vi "Load and Validate_Extract Number.vi"(11 "String":string) -> (3 "Numeric":i32)   [LabVIEW 2020, in "ProjectBuilder.lvlib"]
uses:
  ProjectBuilder.lvlib
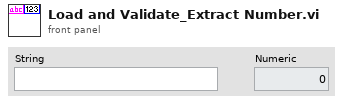
[diagram p1: front panel]
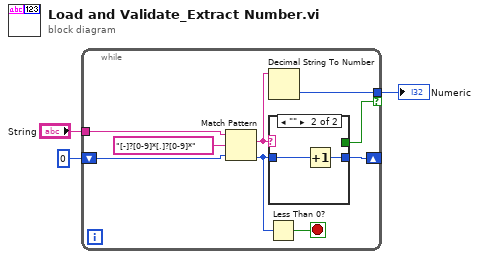
[diagram p0: block diagram]
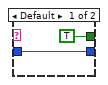
[diagram p2: hidden frame]
diagram:
  n1 = while {
    tunnel: [w12] -> w3 if=w7
    tunnel: "String" -> [w10]
    shift-right: [w6] -> _
    shift-left: 0 -> [w9]
    stop <- w4 stop-if-true
    n2 = Match Pattern(string=w10, regular expression="[-]?[0-9]*[.]?[0-9]*", offset (0)=w9) -> (match substring=w8:string, offset past match=w5:i32)  [unwired: 2 out]
    n3 = Less Than 0?(x=w5) -> (x < 0?=w4:bool)
    n4 = Decimal String To Number(string=w8) -> (number=w12:i32)  [unwired: 2 in, 1 out]
    n5 = case shown="\"\"" w8 {
      tunnel: [w14 w15] -> w6
      tunnel: [TRUE _] -> w7
      tunnel: w5 -> [w14 w16]
      frame Default {
      }
      frame "" {
        n6 = Increment(x=w16) -> (x+1=w15:i32)
      }
    }
  }
  "Numeric" <- w3
